vi "Check Response Status.vi"(8 "Error In":errorcluster, 9 "Body":string, 10 "Headers":string, 11 "Arguments":string[](array[string])) -> (0 "Error Out":errorcluster)   [LabVIEW 2013, in "LVH-XBMC.lvlib"]
uses:
  LVH-XBMC.lvlib
  Type Defs/JSON_Objects/XBMC Error.ctl
  Type Defs/Error.ctl
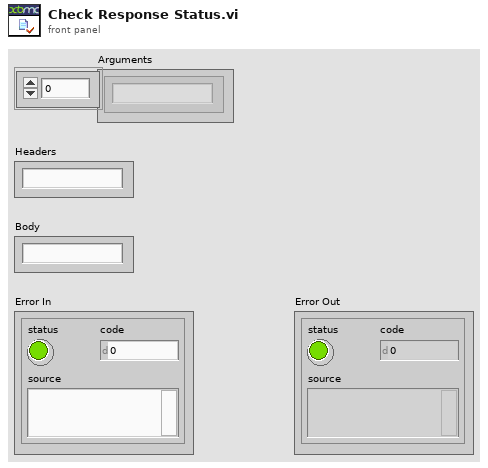
[diagram p1: front panel]
types:
  T1 = typedef "LVH-XBMC.lvlib/Error.ctl" = enum16{"Unauthorized", "XBMC Error"}
  T2 = typedef "LVH-XBMC.lvlib/XBMC Error.ctl" = cluster{"id":dbl, "jsonrpc":string, "error":cluster{"code":dbl, "message":string}}
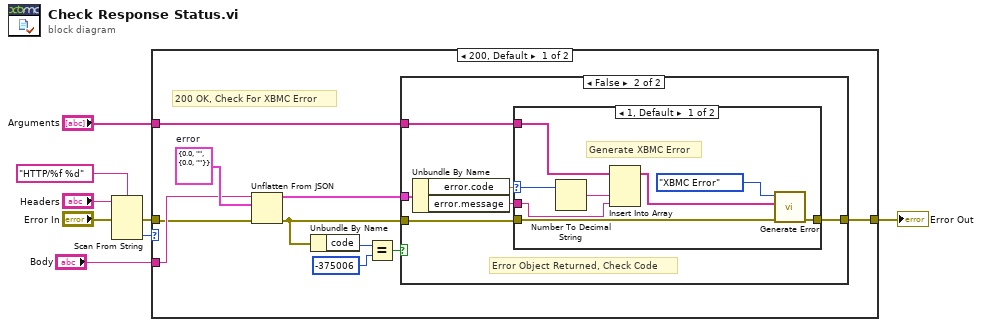
[diagram p0: block diagram]
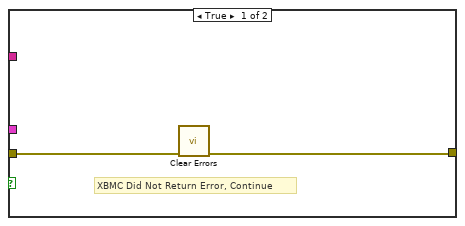
[diagram p2: hidden frame]
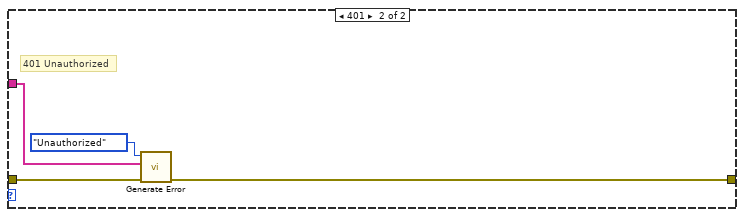
[diagram p4: hidden frame]
diagram:
  n1 = Scan From String(format string="HTTP/%f %d", input string="Headers", error in="Error In") -> (error out=w2:errorcluster, output 2=w4:i32)  [unwired: 4 in, 2 out]
  n2 = case shown="200, Default" w4 {
    tunnel: "Arguments" -> [w14 w37]
    tunnel: [w16 w39] -> w3
    tunnel: w2 -> [w15 w38]
    tunnel: "Body" -> [w17 _]
    frame 200, Default {
      w18 = T2 {"id"=0.0, "jsonrpc"="", "error"={"code"=0.0, "message"=""}}  # error
      # "200 OK, Check For XBMC Error"
      n3 = Unflatten From JSON(JSON string=w17, type and defaults=w18, error in (no error)=w15) -> (value=w13:T2, error out=w10:errorcluster)  [unwired: 4 in]
      n4 = Unbundle By Name(w10) -> ("code"=w11:i32)
      n5 = Equal?(x=w11, y=-375006) -> (x = y?=w12:bool)
      n6 = case shown="False" w12 {
        tunnel: [w19 w26] -> w16
        tunnel: w10 -> [w20 w25]
        tunnel: w14 -> [_ w24]
        tunnel: w13 -> [_ w22]
        frame True {
          # "XBMC Did Not Return Error, Continue"
          n7 = call <vilib>:"Clear Errors.vi"("error in (no error)"=w20) -> ("error out"=w19:errorcluster)  [unwired: 6 in]
        }
        frame False {
          # "Error Object Returned, Check Code"
          n8 = Unbundle By Name(w22) -> ("error.code"=w23:dbl, "error.message"=w21:string)
          n9 = case shown="1, Default" w23 {
            selector: w23 -> [w29 _]
            tunnel: [w32 w35] -> w26
            tunnel: w25 -> [w33 w35]
            tunnel: w24 -> [w31 _]
            tunnel: w21 -> [w27 _]
            frame 1, Default {
              # "Generate XBMC Error"
              n10 = Number To Decimal String(number=w29) -> (decimal integer string=w28:string)  [unwired: 1 in]
              n11 = Insert Into Array(array=w31, new element #1=w28, new element #2=w27) -> (w30:string[])  [unwired: 1 in]
              n12 = call "Generate Error.vi"("Error In"=w33, "Arguments"=w30, "Error"=Error."XBMC Error" ("Enum")) -> ("Error Out"=w32:errorcluster)  [unwired: 8 in]
            }
            frame 0 {
              # "Code = 0, No Error"
            }
          }
        }
      }
    }
    frame 401 {
      # "401 Unauthorized"
      n13 = call "Generate Error.vi"("Error In"=w38, "Arguments"=w37, "Error"=Error."Unauthorized" ("Enum")) -> ("Error Out"=w39:errorcluster)  [unwired: 8 in]
    }
  }
  "Error Out" <- w3
